vi "Read Pin.vi"(8 "error in (no error)":errorcluster, 9 "Pin 2":dbl caption="Pin", 10 "Port 4":dbl caption="Port", 11 "TI in":refnum<class "TI.lvclass">) -> (0 "error out":errorcluster, 3 "TI out":refnum<class "TI.lvclass">)   [LabVIEW 2020, in "TI.lvclass"]
doc: "Read Pin es el vi donde se envian los datos del pin que se desea leer al microcontrolador, se envian los datos de puerto y pin"
uses:
  TI.lvclass
  TI.lvclass/TI.ctl
  20aefec8-dcca-473e-9076-5b465490ea83.vi
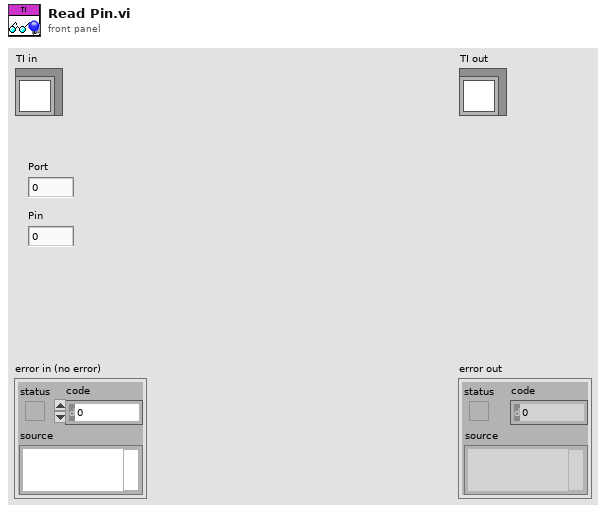
[diagram p1: front panel]
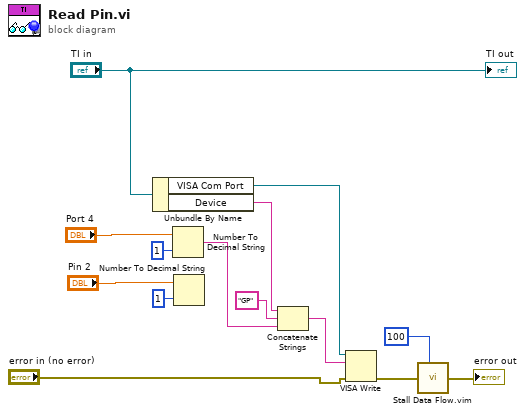
[diagram p0: block diagram]
diagram:
  n1 = Unbundle By Name("TI in") -> ("VISA Com Port"=w13:refnum<visa-resource-name>, "Device"=w11:string)
  n2 = Number To Decimal String(number="Port 4", width (-)=i16 1) -> (decimal integer string=w10:string)
  n3 = Number To Decimal String(number="Pin 2", width (-)=i16 1) -> ()  [unwired: 1 out]
  n4 = Concatenate Strings(w11, "GP" ("string"), w10) -> (w12:string)
  n5 = VISA Write(VISA resource name=w13, write buffer=w12, error in (no error)="error in (no error)") -> (error out=w14:errorcluster)  [unwired: 2 out]
  n6 = call "Stall Data Flow.vim"("value in"=w14, "milliseconds to wait"=u32 100) -> ("value out"=→"error out":errorcluster)  [unwired: 1 out]
  "TI out" <- "TI in"
